vi "PCO_GetBitAlignment.vi"(8 "error in (no error)":errorcluster {"code" format="%x"}, 11 "ph":u64) -> (0 "error out":errorcluster {"code" format="%x"}, 1 "wBitAlignment":u16(ring) items=["BIT_ALIGNMENT_MSB", "BIT_ALIGNMENT_LSB"], 2 "ErrorMessage":i32 format="%x", 3 "ph out":u64)   [LabVIEW 2020, in "SDK.lvlib" / "ImageInformation.lvlib"]
doc: "<b>Description:</b>\nThis function returns the current bit alignment of the transferred image data.\nIf the dynamic resolution of the camera is less than 16 bit/pixel and because the transferred image data is always send as one WORD (16 bit) per pixel, the data can be either MSB or LSB aligned.\n\n<b>Supported camera type:</b>\nAll cameras\n\n<b>Descriptor dependency:</b>\nNone"
uses:
  ImageInformation.lvlib
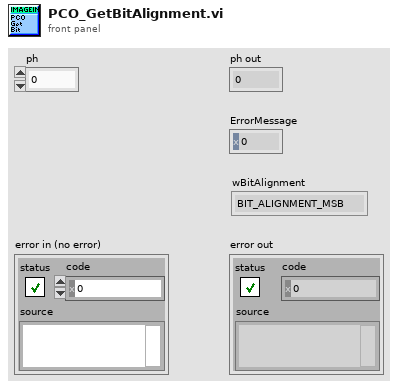
[diagram p1: front panel]
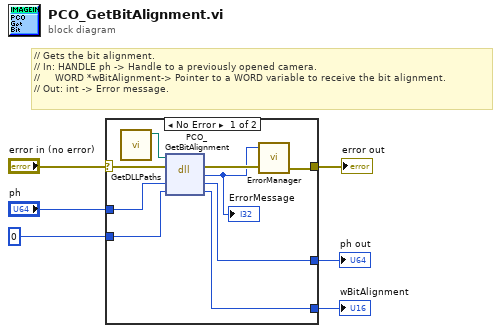
[diagram p0: block diagram]
diagram:
  # "// Gets the bit alignment.\n// In: HANDLE ph -> Handle to a previously opened camera.\n//     WORD *wBitAlignment-> Pointer to a WORD variable to receive the bit alignment.\n// Out: int -> Error message."
  n1 = case shown="No Error" "error in (no error)" {
    selector: "error in (no error)" -> [w11 w18]
    tunnel: "ph" -> [w15 w17]
    tunnel: [w14 w17] -> w5
    tunnel: u16 0 ("wBitAlignment") -> [w13 w16]
    tunnel: [w12 w16] -> w3
    tunnel: [w9 w18] -> w2
    frame No Error {
      n2 = call "GetDLLPaths.vi"() -> ("SC2_Cam_Path"=w7:path)  [unwired: 9 in, 2 out]
      n3 = dll-call lib="?" fn="PCO_GetBitAlignment"(path in=w7, error in=w11, "ph"=w15, "wBitAlignment"=w13) -> (error out=w10:errorcluster, "return type"=w8:i32, "ph"=w14:u64, "wBitAlignment"=w12:u16)  [unwired: 1 in, 1 out]
      "ErrorMessage" <- w8
      n4 = call "ErrorManager.vi"("error in (no error)"=w10, "error code"=w8) -> ("error out"=w9:errorcluster)  [unwired: 3 in]
    }
    frame Error {
    }
  }
  "ph out" <- w5
  "wBitAlignment" <- w3
  "error out" <- w2
